vi "Get Count.vi"(8 "error in (no error)":errorcluster, 11 "Reversi in":refnum<class "Reversi.lvclass">) -> (0 "error out":errorcluster, 1 "Count of White":i16, 2 "Count of Black":i16, 3 "Reversi out":refnum<class "Reversi.lvclass">)   [LabVIEW 2020, in "Reversi.lvlib" / "Reversi.lvclass"]
uses:
  Reversi.lvclass
  Space Ring.ctl
  Reversi.lvclass/Reversi.ctl
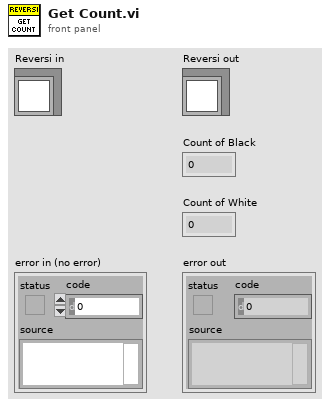
[diagram p1: front panel]
types:
  T1 = typedef "Reversi.lvlib/Reversi.lvclass/Space Ring.ctl" = u16
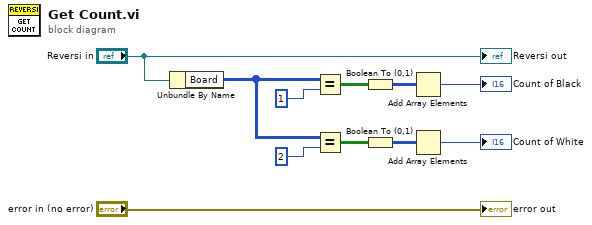
[diagram p0: block diagram]
diagram:
  n1 = Unbundle By Name("Reversi in") -> ("Board"=w2:T1[][])
  n2 = Equal?(x=w2, y=T1 1 ("Space Ring")) -> (x = y?=w8:bool[][])
  n3 = Equal?(x=w2, y=T1 2 ("Space Ring")) -> (x = y?=w4:bool[][])
  n4 = Boolean To (0,1)(Boolean=w8) -> (0, 1=w7:i16[][])
  n5 = Boolean To (0,1)(Boolean=w4) -> (0, 1=w5:i16[][])
  n6 = Add Array Elements(numeric array=w7) -> (sum=→"Count of Black":i16)
  n7 = Add Array Elements(numeric array=w5) -> (sum=→"Count of White":i16)
  "error out" <- "error in (no error)"
  "Reversi out" <- "Reversi in"
